vi "wrie-ref-istance.vi"(8 "error in (no error)":errorcluster, 10 "dbc.data":refnum<data-value>, 11 "dbc in":refnum<class "dbc.lvclass">) -> (0 "error out":errorcluster, 3 "dbc out":refnum<class "dbc.lvclass">)   [LabVIEW 2015, in "dbc.lvclass"]
uses:
  dbc.lvclass
  controls/dbc-file-data.ctl
  dbc.lvclass/dbc.ctl
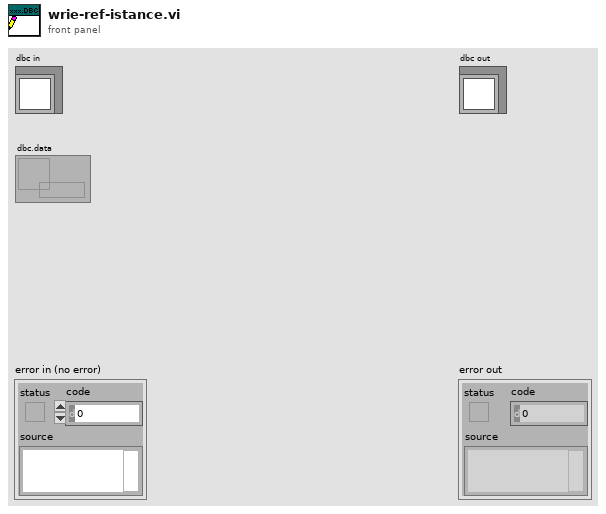
[diagram p1: front panel]
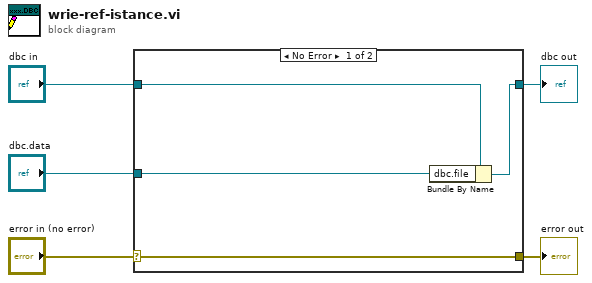
[diagram p0: block diagram]
diagram:
  n1 = case shown="No Error" "error in (no error)" {
    selector: "error in (no error)" -> [w9 w10]
    tunnel: [w9 w10] -> w4
    tunnel: [w7 w11] -> w2
    tunnel: "dbc in" -> [w8 w11]
    tunnel: "dbc.data" -> [w6 _]
    frame No Error {
      n2 = Bundle By Name(cluster=w8, "dbc.file"=w6) -> (w7:refnum<class "dbc.lvclass">)
    }
    frame Error {
    }
  }
  "error out" <- w4
  "dbc out" <- w2
